vi "SRV_System Config GUI.vi"(11 "System Config File Path in":path) -> (0 "error out":errorcluster, 1 "Cancelled?":bool, 3 "System Config Filepath":path)   [LabVIEW 2009]
doc: "A Producer-Consumer two-loop state machine template. This template uses the LPD Command Queues to drive its execution.\n\nThere are several advantages such as:\n- convenient error state control\n- the ability to pass data between states/loops/VIs via a variant\n- command history which is extremely valuable in troubleshooting when an error occurs\n\n\nAuthor: Mike Schultz\n\nLogicPD, Inc\nwww.logicpd.com"
uses:
  SRV_System Config.ctl
  Watchdog/SRV_Watchdog Config Cluster.ctl
  Motors/Motors Config/SRV_Motor Control Command Config.ctl
  Support/SRV_Command-Data Queue Data Type.ctl
panel:
  in  "System Config":T1={"SRV IP Address"="", "Video Stream Rate Period (ms)"=250, "Enable Diagnostic Log"=FALSE, "Watchdog 1 Config"={"Watchdog Name"="", "Watchdog Period (s)"=1.0, "Watchdog Command"={"I2C Address"=0, "Register"=0, "Value"=0, "Active"=FALSE}}, "Watchdog 2 Config"={"Watchdog Name"="", "Watchdog Period (s)"=1.0, "Watchdog Command"={"I2C Address"=0, "Register"=0, "Value"=0, "Active"=FALSE}}, "Sensor Window Filepath"=path ""} {"Watchdog 2 Config"."Watchdog Period (s)" format="%.3f"; "Watchdog 2 Config"."Watchdog Command"."Value" format="%02x"; "Watchdog 2 Config"."Watchdog Command"."Register" format="%02x"; "Watchdog 2 Config"."Watchdog Command"."I2C Address" format="%02x"; "Watchdog 1 Config"."Watchdog Period (s)" format="%.3f"; "Watchdog 1 Config"."Watchdog Command"."Value" format="%02x"; "Watchdog 1 Config"."Watchdog Command"."Register" format="%02x"; "Watchdog 1 Config"."Watchdog Command"."I2C Address" format="%02x"; "Video Stream Rate Period (ms)" min=33 max=10000 step=1}
  in  "Cancel Button":bool
  in  "OK Button":bool
  in  "About":bool
  # "I2C Address"
  # "Register"
  # "Value"
  # "Active"
  # "I2C Address"
  # "Register"
  # "Value"
  # "Active"
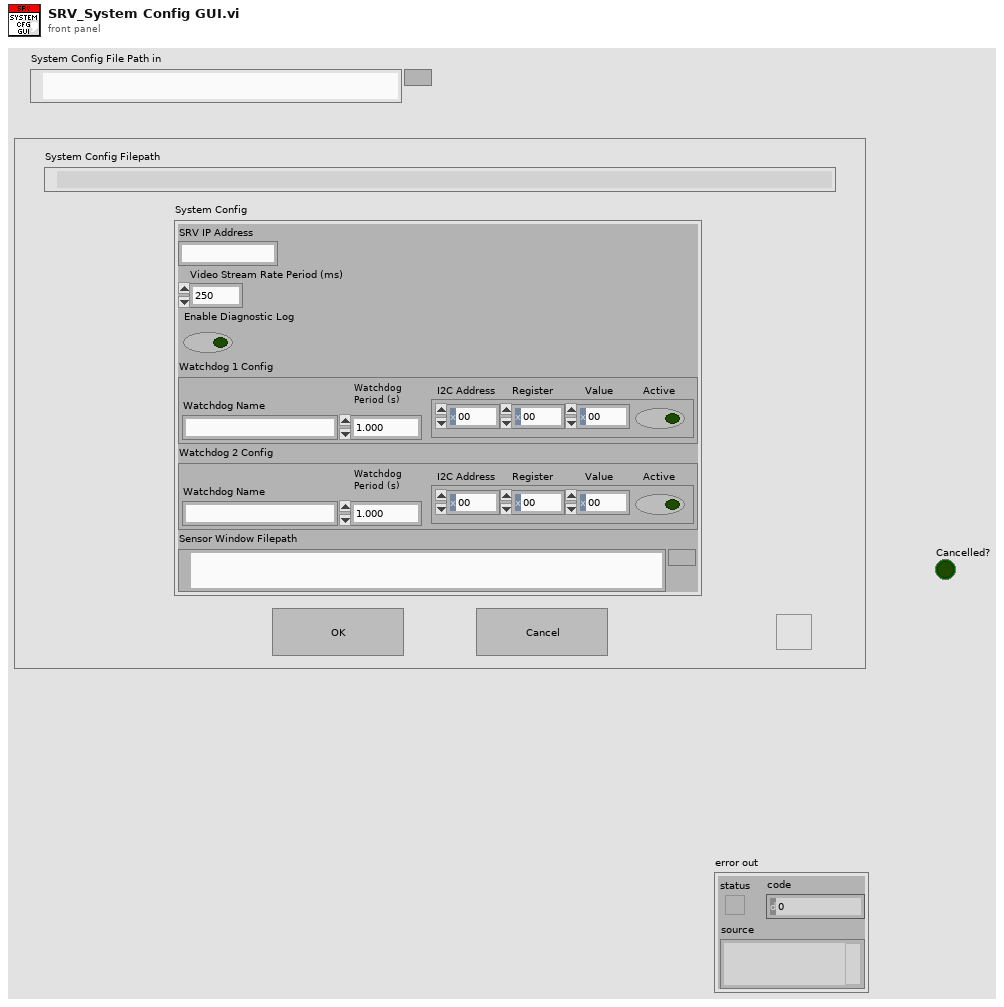
[diagram p1: front panel]
types:
  T1 = typedef "SRV_System Config.ctl" = cluster{"SRV IP Address":string, "Video Stream Rate Period (ms)":u32, "Enable Diagnostic Log":bool, "Watchdog 1 Config":T2, "Watchdog 2 Config":T2, "Sensor Window Filepath":path}
  T2 = typedef "SRV_Watchdog Config Cluster.ctl" = cluster{"Watchdog Name":string, "Watchdog Period (s)":dbl, "Watchdog Command":T3}
  T3 = typedef "SRV_Motor Control Command Config.ctl" = cluster{"I2C Address":u8, "Register":u8, "Value":u8, "Active":bool}
  T4 = typedef "SRV_Command-Data Queue Data Type.ctl" = cluster{"Command":string, "Data":variant}
  T5 = cluster{"user event":refnum<user-event>, "System Config Filepath":path, "System Config":T1, "Cancelled?":bool}
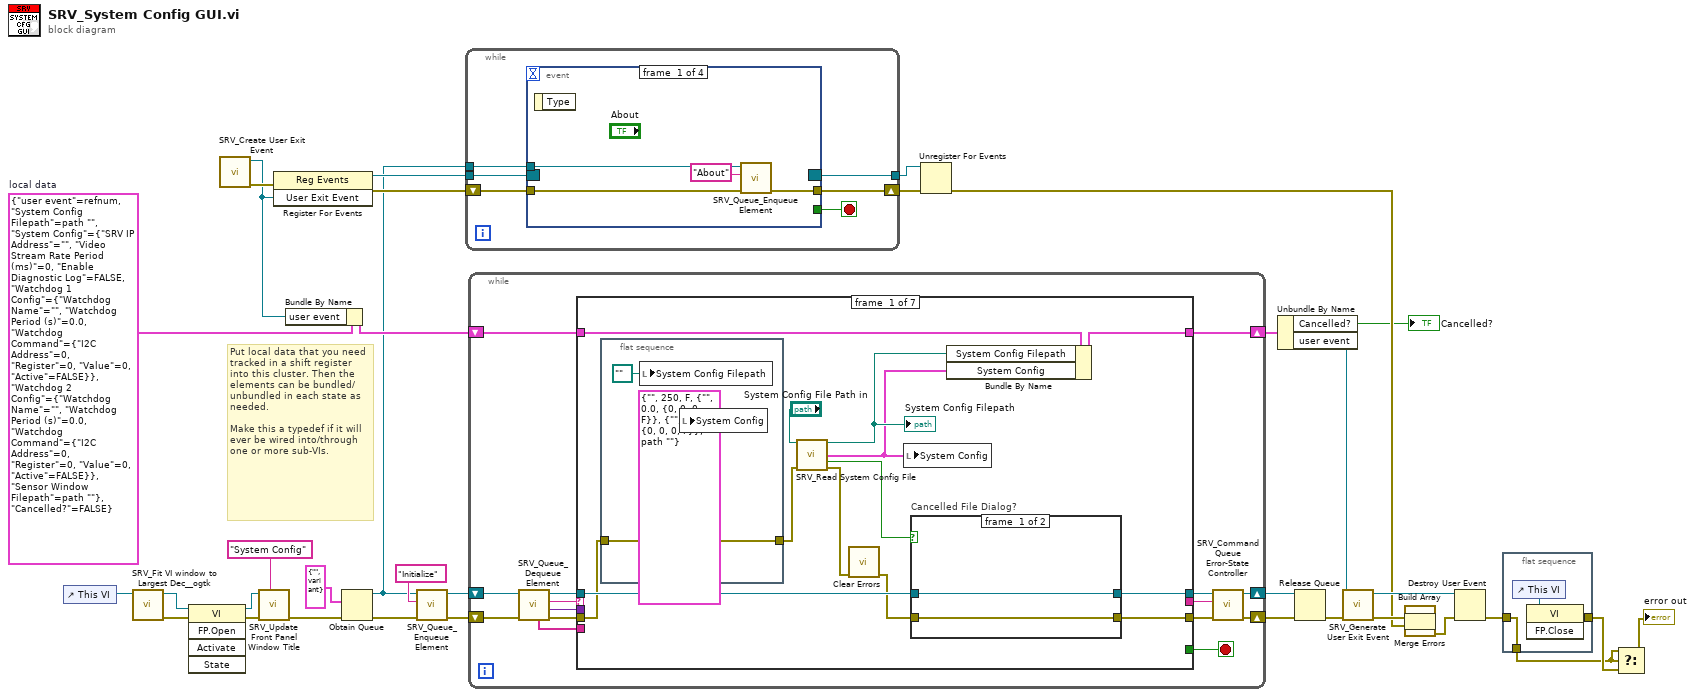
[diagram p0: block diagram]
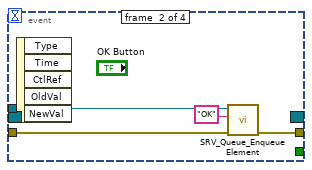
[diagram p2: hidden frame]
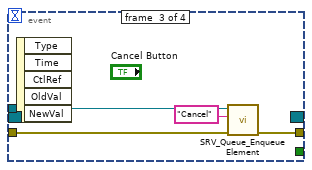
[diagram p3: hidden frame]
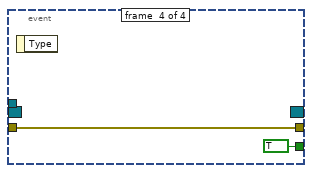
[diagram p4: hidden frame]
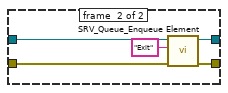
[diagram p5: hidden frame]
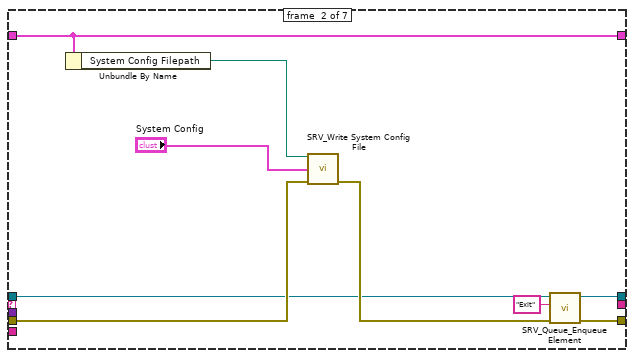
[diagram p6: hidden frame]
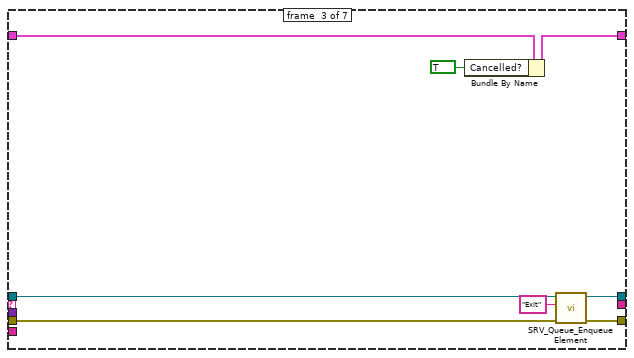
[diagram p7: hidden frame]
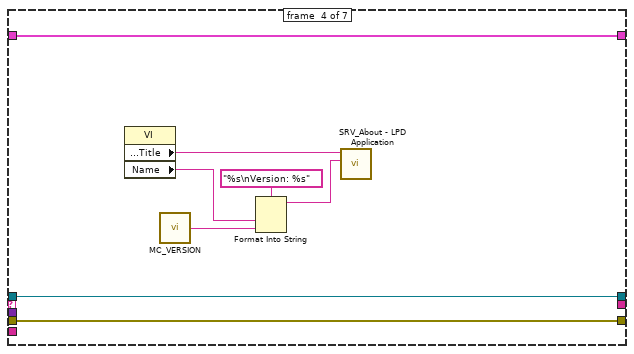
[diagram p8: hidden frame]
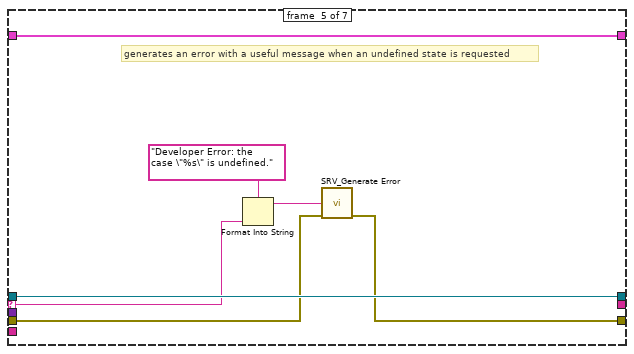
[diagram p9: hidden frame]
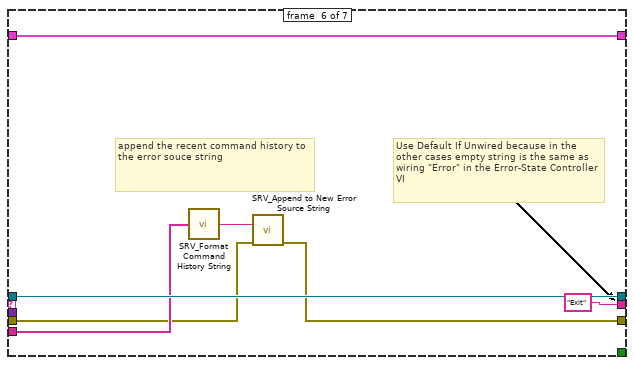
[diagram p10: hidden frame]
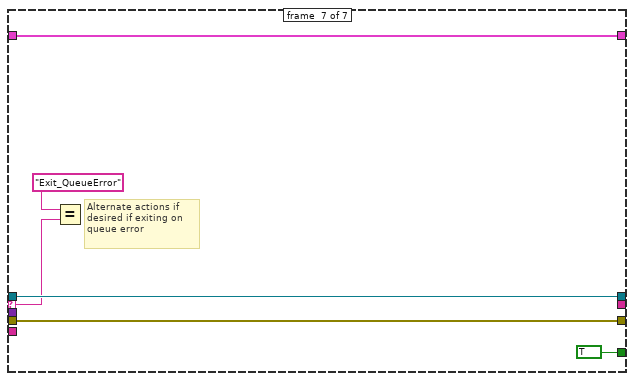
[diagram p11: hidden frame]
diagram:
  w30 = T5 {"user event"=refnum, "System Config Filepath"=path "", "System Config"={"SRV IP Address"="", "Video Stream Rate Period (ms)"=0, "Enable Diagnostic Log"=FALSE, "Watchdog 1 Config"={"Watchdog Name"="", "Watchdog Period (s)"=0.0, "Watchdog Command"={"I2C Address"=0, "Register"=0, "Value"=0, "Active"=FALSE}}, "Watchdog 2 Config"={"Watchdog Name"="", "Watchdog Period (s)"=0.0, "Watchdog Command"={"I2C Address"=0, "Register"=0, "Value"=0, "Active"=FALSE}}, "Sensor Window Filepath"=path ""}, "Cancelled?"=FALSE}  # local data
  # "Put local data that you need tracked in a shift register into this cluster. Then the elements can be bundled/unbundled in each state as needed.\n\nMake this a typedef if it will ever be wired into/through one or more sub-VIs."
  n1 = control-ref of="This VI"() -> (w6:refnum<vi>)
  n2 = call "SRV_Fit VI window to Largest Dec__ogtk.vi"("VI Ref (calling VI)"=w6) -> ("error out"=w8:errorcluster, "dup VI Ref"=w5:refnum<vi>)  [unwired: 5 in]
  n3 = invoke class="VI" method="FP.Open"(reference=w5, error in=w8) -> (reference out=w1:refnum<vi>, error out=w3:errorcluster)  [unwired: 3 in, 3 out]
  n4 = call "SRV_Create User Exit Event.vi"() -> ("error out"=w21:errorcluster, "User Exit Event"=w20:refnum<user-event>)  [unwired: 10 in]
  n5 = call "SRV_Update Front Panel Window Title.vi"("Window Title Override String"="System Config", "error in (no error)"=w3, "VI ref"=w1) -> ("error out"=w2:errorcluster)  [unwired: 7 in, 1 out]
  n6 = register-events(error in=w21, w20) -> (reference out=w36:refnum<event-registration>, error out=w35:errorcluster)  [unwired: 1 in]
  n7 = Bundle By Name(cluster=w30, "user event"=w20) -> (w29:T5)
  n8 = Obtain Queue(element data type=T4 {"Command"="", "Data"=variant} ("Queue Data Type"), error in (no error)=w2) -> (queue out=w16:refnum<queue>, error out=w17:errorcluster)  [unwired: 3 in, 1 out]
  n9 = call "SRV_Queue_Enqueue Element.vi"("error in (no error)"=w17, "Command"="Initialize", "Command-Data Queue"=w16) -> ("error out"=w13:errorcluster, "Command-Data Queue out"=w15:refnum<queue>)  [unwired: 6 in, 1 out]
  n10 = while {
    shift-right: [w41] -> w33
    shift-left: w35 -> [w42]
    tunnel: w16 -> [w40]
    tunnel: w36 -> [w39]
    tunnel: [w38] -> w34
    stop <- w37 stop-if-true
    n11 = event shown="[2] \"Cancel Button\": Value Change" {
      selector: w39 -> [_ _ _ _]
      dyn-events: [_ _ _ _] -> w38
      timeout: _ -> [_ _ _ _]
      tunnel: w42 -> [w46 w48 w52 w56]
      tunnel: [w45 w49 w53 w56] -> w41
      tunnel: w40 -> [w43 w47 w51 _]
      tunnel: [_ _ _ TRUE] -> w37
      event #0 {
        n12 = event-data() -> ()  [unwired: 1 in, 1 out]
        n13 = call "SRV_Queue_Enqueue Element.vi"("error in (no error)"=w46, "Command"="About", "Command-Data Queue"=w43) -> ("error out"=w45:errorcluster)  [unwired: 6 in, 2 out]
      }
      event #1 {
        n14 = event-data() -> ()  [unwired: 1 in, 5 out]
        n15 = call "SRV_Queue_Enqueue Element.vi"("error in (no error)"=w48, "Command"="OK", "Command-Data Queue"=w47) -> ("error out"=w49:errorcluster)  [unwired: 6 in, 2 out]
      }
      event #2 {
        n16 = event-data() -> ()  [unwired: 1 in, 5 out]
        n17 = call "SRV_Queue_Enqueue Element.vi"("error in (no error)"=w52, "Command"="Cancel", "Command-Data Queue"=w51) -> ("error out"=w53:errorcluster)  [unwired: 6 in, 2 out]
      }
      event #3 {
        n18 = event-data() -> ()  [unwired: 1 in, 1 out]
      }
    }
  }
  n19 = while {
    shift-right: [w65] -> w32
    shift-left: w13 -> [w71]
    shift-right: [w63] -> w31
    shift-left: w15 -> [w69]
    shift-right: [w57] -> w28
    shift-left: w29 -> [w58]
    stop <- w59 stop-if-true
    n20 = call "SRV_Queue_Dequeue Element.vi"("error in (no error)"=w71, "Command-Data Queue"=w69) -> ("error out"=w70:errorcluster, "Data"=w62:variant, "Command"=w67:string, "Command-Data Queue out"=w68:refnum<queue>, "Command History"=w61:string[])  [unwired: 4 in, 1 out]
    n21 = case shown="\"About\"" w67 {
      selector: w67 -> [_ _ _ _ w124 _ w136]
      tunnel: w70 -> [w76 w101 w110 w118 w122 w128 w138]
      tunnel: [w82 w98 w109 w118 w121 w129 w138] -> w66
      tunnel: w68 -> [w83 w97 w111 w119 w126 w133 w139]
      tunnel: [w81 w96 w108 w119 w126 w133 w139] -> w64
      tunnel: w62 -> [_ _ _ _ _ _ _]
      tunnel: w61 -> [_ _ _ _ _ w132 _]
      tunnel: [_ _ _ _ _ "Exit" ("Error Command") _] -> w60
      tunnel: [_ _ _ _ _ _ TRUE] -> w59
      tunnel: w58 -> [w80 w103 w106 w113 w123 w130 w134]
      tunnel: [w79 w103 w105 w113 w123 w130 w134] -> w57
      frame #0 {
        n22 = flat-sequence {
          tunnel: [w86] -> w77
          tunnel: w76 -> [w86]
          frame #0 {
            n23 = local write "System Config Filepath"(path "" ("Sensor Config Filepath")) -> ()
            n24 = local write "System Config"(T1 {"SRV IP Address"="", "Video Stream Rate Period (ms)"=250, "Enable Diagnostic Log"=FALSE, "Watchdog 1 Config"={"Watchdog Name"="", "Watchdog Period (s)"=0.0, "Watchdog Command"={"I2C Address"=0, "Register"=0, "Value"=0, "Active"=FALSE}}, "Watchdog 2 Config"={"Watchdog Name"="", "Watchdog Period (s)"=0.0, "Watchdog Command"={"I2C Address"=0, "Register"=0, "Value"=0, "Active"=FALSE}}, "Sensor Window Filepath"=path ""} ("System Config")) -> ()
          }
        }
        n25 = call "SRV_Read System Config File.vi"("System Config File Path"="System Config File Path in", "error in (no error)"=w77) -> ("System Config File Path out"=w78:path, "System Config"=w75:T1, "Cancelled?"=w84:bool, "error out"=w73:errorcluster)  [unwired: 10 in]
        "System Config Filepath" <- w78
        n26 = call <vilib>:"Clear Errors.vi"("error in (no error)"=w73) -> ("error out"=w72:errorcluster)  [unwired: 6 in]
        n27 = local write "System Config"(w75) -> ()
        n28 = case "Cancelled File Dialog?" shown="True" w84 {
          tunnel: w72 -> [w88 w93]
          tunnel: w83 -> [w89 w94]
          tunnel: [w88 w92] -> w82
          tunnel: [w89 w91] -> w81
          frame #0 {
          }
          frame #1 {
            n29 = call "SRV_Queue_Enqueue Element.vi"("error in (no error)"=w93, "Command"="Exit", "Command-Data Queue"=w94) -> ("error out"=w92:errorcluster, "Command-Data Queue out"=w91:refnum<queue>)  [unwired: 6 in, 1 out]
          }
        }
        n30 = Bundle By Name(cluster=w80, "System Config Filepath"=w78, "System Config"=w75) -> (w79:T5)
      }
      frame #1 {
        n31 = Unbundle By Name(w103) -> ("System Config Filepath"=w102:path)
        n32 = call "SRV_Write System Config File.vi"("System Config File Path"=w102, "System Config"="System Config", "error in (no error)"=w101) -> ("error out"=w99:errorcluster)  [unwired: 12 in]
        n33 = call "SRV_Queue_Enqueue Element.vi"("error in (no error)"=w99, "Command"="Exit", "Command-Data Queue"=w97) -> ("error out"=w98:errorcluster, "Command-Data Queue out"=w96:refnum<queue>)  [unwired: 6 in, 1 out]
      }
      frame #2 {
        n34 = Bundle By Name(cluster=w106, "Cancelled?"=TRUE) -> (w105:T5)
        n35 = call "SRV_Queue_Enqueue Element.vi"("error in (no error)"=w110, "Command"="Exit", "Command-Data Queue"=w111) -> ("error out"=w109:errorcluster, "Command-Data Queue out"=w108:refnum<queue>)  [unwired: 6 in, 1 out]
      }
      frame #3 {
        n36 = property class="VI"() -> ("Front Panel.Title"=w117:string, "Name"=w114:string)  [unwired: 2 in, 2 out]
        n37 = call "MC_VERSION.vi"() -> ("MC Version"=w112:string)
        n38 = Format Into String(format string="%s\nVersion: %s", w114, w112) -> (resulting string=w115:string)  [unwired: 2 in, 1 out]
        n39 = call "SRV_About - LPD Application.vi"("Version Info"=w115, "Application Name"=w117) -> ()  [unwired: 10 in]
      }
      frame #4 {
        # "generates an error with a useful message when an undefined state is requested"
        n40 = Format Into String(format string="Developer Error: the case \"%s\" is undefined.", w124) -> (resulting string=w120:string)  [unwired: 2 in, 1 out]
        n41 = call "SRV_Generate Error.vi"("Message"=w120, "error in (no error)"=w122) -> ("error out"=w121:errorcluster)  [unwired: 13 in]
      }
      frame #5 {
        # "Use Default If Unwired because in the other cases empty string is the same as wiring \"Error\" in the Error-State Controller VI"
        # "append the recent command history to the error souce string"
        n42 = call "SRV_Format Command History String.vi"("Command History"=w132) -> ("Command History String"=w127:string)  [unwired: 14 in]
        n43 = call "SRV_Append to New Error Source String.vi"("Message String to append"=w127, "Error In (no error)"=w128) -> ("error out"=w129:errorcluster)  [unwired: 13 in]
      }
      frame #6 {
        # "Alternate actions if desired if exiting on queue error"
        n44 = Equal?(x="Exit_QueueError", y=w136) -> ()  [unwired: 1 out]
      }
    }
    n45 = call "SRV_Command Queue Error-State Controller.vi"("error in (no error)"=w66, "Error Command"=w60, "Command-Data Queue"=w64) -> ("error out"=w65:errorcluster, "Command-Data Queue out"=w63:refnum<queue>)  [unwired: 7 in]
  }
  n46 = Unregister For Events(event registration refnum=w34, error in=w33) -> (error out=w23:errorcluster)
  n47 = Unbundle By Name(w28) -> ("Cancelled?"=→"Cancelled?":bool, "user event"=w27:refnum<user-event>)
  n48 = Release Queue(queue=w31, error in (no error)=w32) -> (error out=w26:errorcluster)  [unwired: 1 in, 2 out]
  n49 = call "SRV_Generate User Exit Event.vi"("error in (no error)"=w26, "User Exit Event"=w27) -> ("error out"=w24:errorcluster, "User Exit Event out"=w25:refnum<user-event>)  [unwired: 8 in]
  n50 = Build Array(w24, w23) -> (w19:errorcluster[])
  n51 = call <vilib>:"Merge Errors.vi"("error array in"=w19) -> ("error out"=w22:errorcluster)  [unwired: 6 in]
  n52 = Destroy User Event(user event=w25, error in=w22) -> (error out=w10:errorcluster)
  n53 = flat-sequence {
    tunnel: [w141] -> w12
    tunnel: w10 -> [w140]
    tunnel: [w140] -> w9
    frame #0 {
      n54 = control-ref of="This VI"() -> (w142:refnum<vi>)
      n55 = invoke class="VI" method="FP.Close"(reference=w142) -> (error out=w141:errorcluster)  [unwired: 2 in, 2 out]
    }
  }
  n56 = Select(t=w9, s=w9, f=w12) -> (s? t:f=→"error out":errorcluster)
